vi "HideUnusedControls.vi"(11 "AllControlsRefs":T22) -> ()   [LabVIEW 2013]
uses:
  <instrlib>/DG535/Command/DG535_TriggerMode.ctl
  <instrlib>/DG535/SRS_DG535_Lib.lvlib
  <instrlib>/DG535/Command/DG535_Output.ctl
  <instrlib>/DG535/Command/DG535_Channel.ctl
  <instrlib>/DG535/Command/Set Output.ctl
  <instrlib>/DG535/Command/Set Delay.ctl
  <instrlib>/DG535/Command/Set Trigger.ctl
  ControlDef/AllControlsRefs.ctl
  ControlDef/ProcessingMode.ctl
  <instrlib>/AnalogDiscSDKLv/VIs/DWF_TrigSrc.ctl
  <instrlib>/AnalogDiscSDKLv/AnalogDiscSDKLv.lvlib
  <instrlib>/AnalogDiscSDKLv/VIs/DWF_Filter.ctl
  <instrlib>/AnalogDiscSDKLv/VIs/DWF_AcqMode.ctl
  <instrlib>/AnalogDiscSDKLv/VIs/DWF_TrigCond.ctl
  <instrlib>/AnalogDiscSDKLv/VIs/DWF_TrigType.ctl
  <instrlib>/AnalogDiscSDKLv/VIs/DWF_AnalogIn_Configurations.ctl
  <instrlib>/GageLv_uic/VI/Gage_Configs.ctl
  <instrlib>/GageLv_uic/Gage.lvlib
  ControlDef/InstruMode_Typedef.ctl
  ControlDef/LaserCtrl_Method.ctl
  ControlDef/MainDAQ_Selector.ctl
panel:
  in  "InstruConfig":T18 {"DG535"."Trigger"."External  Level" min=-2.56 max=2.56 format="%.2f"; "DG535"."Trigger"."Internal/Burst Rate" min=0.001 max=1000000.0 format="%.3f"; "DG535"."Delays"."Delay" format="%#_6p"; "DG535"."Output"."Offset" min=-3.0 max=4.0 format="%.2f"; "DG535"."Output"."Amplitude" min=-3.0 max=4.0 format="%.2f"; "Gage_Config"."Trigger"."External Impedance" items=["50 Ohm", "HiZ"]; "Gage_Config"."Trigger"."External Coupling" items=["DC", "AC"]; "Gage_Config"."Trigger"."External Range" min=2000 max=10000 step=8000; "Gage_Config"."Trigger"."Slope" items=["Rising", "Falling"]; "Gage_Config"."Trigger"."Level" min=-100 max=100; "Gage_Config"."Trigger"."Source" min=0 max=64 step=1; "Gage_Config"."Channels"."Impedance" min=50 max=1000000 step=999950; "Gage_Config"."Channels"."Coupling" items=["DC", "AC"]; "Gage_Config"."Acquisition"."Segment Size" min=256.0 step=128.0; "Gage_Config"."Acquisition"."Trigger Delay" min=0.0 step=128.0; "Gage_Config"."Acquisition"."Trigger Timeout" format="%.0p"; "Gage_Config"."Acquisition"."Trigger Holdoff" min=0.0 step=128.0; "Gage_Config"."Acquisition"."Depth" min=256.0 step=128.0; "Gage_Config"."Acquisition"."Mode" items=["Single", "Dual", "Quad", "Octal"]; "Gage_Config"."Acquisition"."Sample Rate" format="%.0p"; "AnalogDisc_Config"."AnalogTrigger"."Level(V)" format="%#_6p"; "AnalogDisc_Config"."AnalogTrigger"."Hysterisis(V)" format="%#_6p"; "AnalogDisc_Config"."Acqusition"."RecordLength(s)" format="%#_6p"; "AnalogDisc_Config"."Acqusition"."Freq(Hz,SampleRate)" format="%#_6p"; "AnalogDisc_Config"."Trigger"."Position/Delay(s)" format="%#_6p"; "AnalogDisc_Config"."Trigger"."Holdoff(s)" format="%#_6p"; "AnalogDisc_Config"."Trigger"."Timeout(s)" format="%#_6p"}
  in  "DG535_Configs":T19={"Trigger"={"Trigger Mode"=enum."External", "Internal/Burst Rate"=10.0, "External  Level"=1.5, "Impedance"=TRUE, "Slope"=FALSE}, "Delays"=[{"Channel"=enum."A Output", "Sync To"=enum."T0 Output", "Delay"=0.099807701}, {"Channel"=enum."B Output", "Sync To"=enum."A Output", "Delay"=1.2e-05}, {"Channel"=enum."C Output", "Sync To"=enum."T0 Output", "Delay"=0.0}, {"Channel"=enum."D Output", "Sync To"=enum."T0 Output", "Delay"=1e-05}, {"Channel"=enum."Trigger Input", "Sync To"=enum."T0 Output", "Delay"=0.0}], "Output"=[{"Channel"=enum."A Output", "Level"=enum."TTL", "Load"=TRUE, "Polarity"=FALSE, "Amplitude"=1.0, "Offset"=0.0}, {"Channel"=enum."B Output", "Level"=enum."TTL", "Load"=FALSE, "Polarity"=TRUE, "Amplitude"=1.0, "Offset"=0.0}, {"Channel"=enum."C Output", "Level"=enum."TTL", "Load"=TRUE, "Polarity"=FALSE, "Amplitude"=1.0, "Offset"=0.0}, {"Channel"=enum."D Output", "Level"=enum."TTL", "Load"=TRUE, "Polarity"=FALSE, "Amplitude"=1.0, "Offset"=0.0}, {"Channel"=enum."T0 Output", "Level"=enum."TTL", "Load"=FALSE, "Polarity"=FALSE, "Amplitude"=1.0, "Offset"=0.0}, {"Channel"=enum."AB Output", "Level"=enum."TTL", "Load"=TRUE, "Polarity"=FALSE, "Amplitude"=1.0, "Offset"=0.0}, {"Channel"=enum."CD Output", "Level"=enum."TTL", "Load"=TRUE, "Polarity"=FALSE, "Amplitude"=1.0, "Offset"=0.0}]} caption="DG535 Settings (Restart Needed)" {"Trigger"."External  Level" min=-2.56 max=2.56 format="%.2f"; "Trigger"."Internal/Burst Rate" min=0.001 max=1000000.0 format="%.3f"; "Delays"."Delay" format="%#_6p"; "Output"."Offset" min=-3.0 max=4.0 format="%.2f"; "Output"."Amplitude" min=-3.0 max=4.0 format="%.2f"}
  in  "SRS On/Off":bool caption="Dont Rely On\nShowing\nCheck BNC"
  in  "Internal/Burst Rate":dbl=10.0 caption="Internal/Burst Rate (Hz)" min=0.001 max=1000000.0 format="%.3f"
  in  "Trigger Mode (SRS)":T5=enum."External" caption="Trigger Mode"
  in  "Ch_D":dbl=2.8e-05 format="%_3ps"
  in  "Ch_C":dbl format="%_3ps"
  in  "Ch_B":dbl=3e-05 format="%_3ps"
  in  "Ch_A":dbl=0.099807701 format="%_3ps"
  in  "Delay A":dbl format="%_3ps"
  in  "Width B":dbl=1e-06 min=0.0 max=9.9e-05 step=1e-09 format="%_3ps"
  in  "Width A":dbl=1e-06 min=0.0 max=9.9e-05 step=1e-09 format="%_3ps"
  in  "Delay B":dbl min=0.0 max=9.9e-05 step=1e-09 format="%_3ps"
  in  "Rep.Rate (BNC)":dbl=10.0 caption="Repetive Rate" min=0.0 max=1000.0 format="%#_6f Hz"
  in  "Mode (BNC)":T20(ring)=enum."Single Shot" caption="Mode"
  in  "Channels Enable Status":bool[](array[boolean])=[TRUE, TRUE]
  in  "Trigger Mode (BNC)":T21(ring)=enum."Triggered" caption="Trigger Mode"
  in  "BNC On/Off":bool caption="Dont Rely On\nShowing\nCheck BNC"
  in  "ManlTrig(SDG)":bool caption="Manual Trigger"
  in  "Mode(SDG_II)":bool caption="Mode"
  in  "Switch(SDG_II)":bool caption="Status"
  out "Nd:YAG Energy":dbl(slide) caption="Nd:YAG Energy (J)" scale=0.0..0.03 scale format="%#_2p"
  out "High Voltages":T23 {"Einzel (Source)" format="%#.0f"; "Einzel (TOF)" format="%#.0f"; "Cone" format="%#.0f"}
  out "LaserEnergy":dbl(slide) caption="Spitfire Energy (J)" scale=0.0..2e-06 scale format="%#_2p"
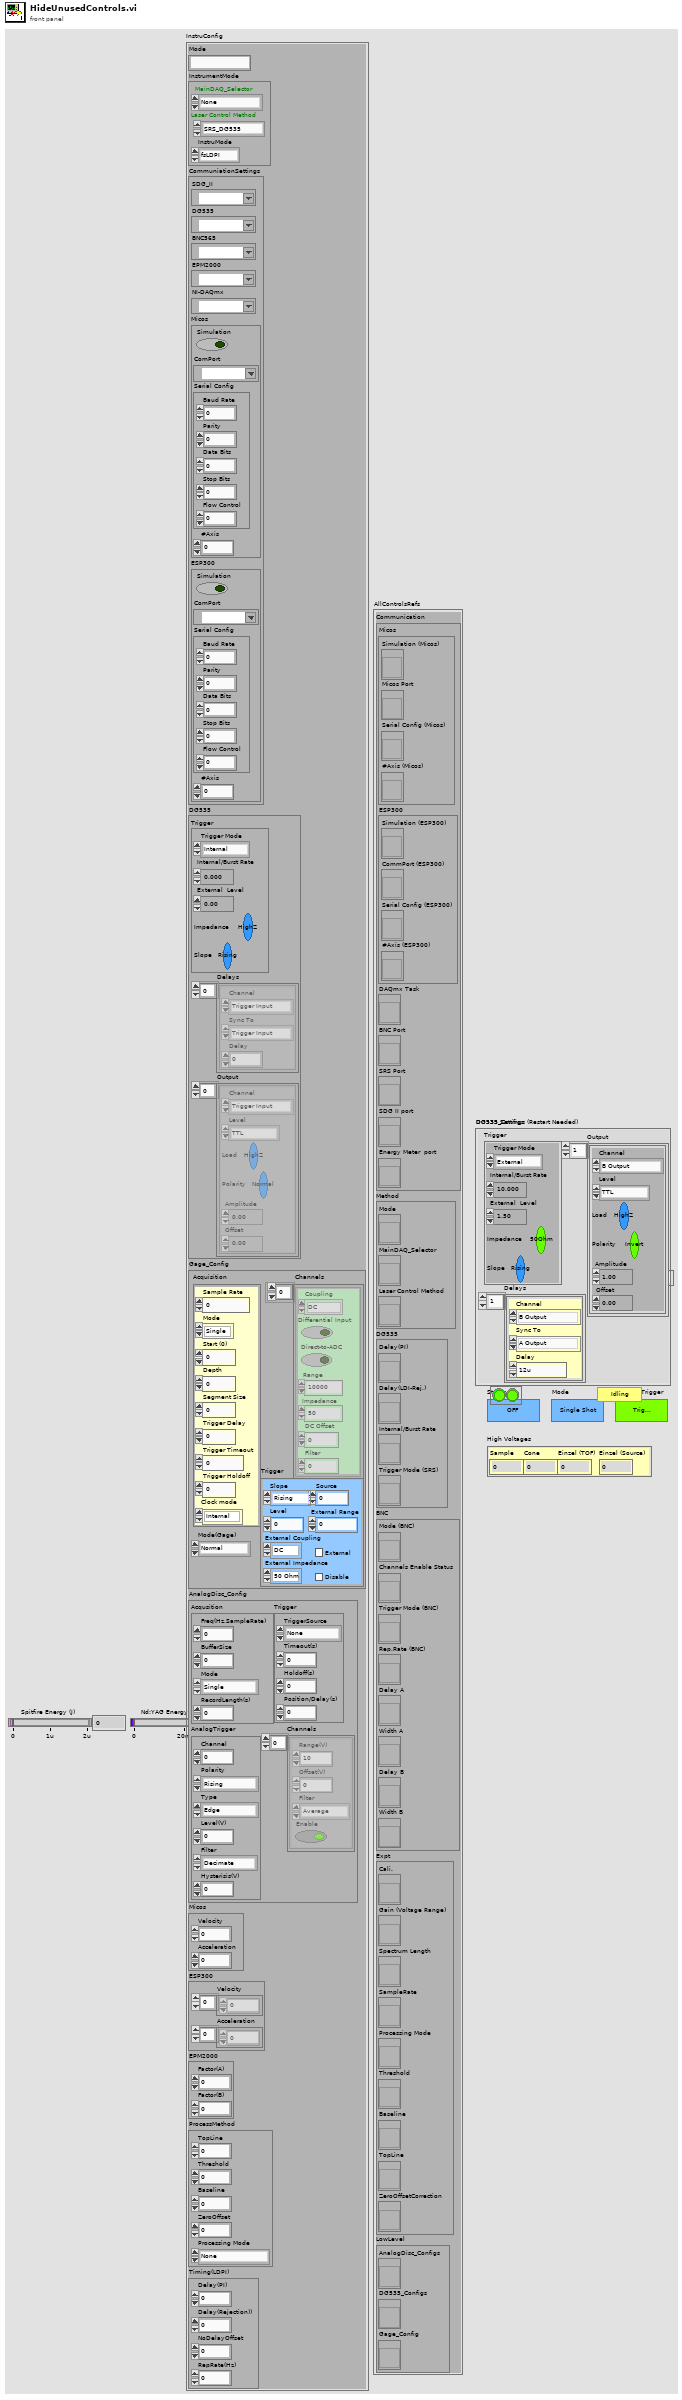
[diagram p1: front panel]
types:
  T1 = typedef "MainDAQ_Selector.ctl" = enum16{"None", "Gage", "Gage_Double", "IonWerks_TDCx4", "Tektronics", "KnifeEdge_Emu", "AnalogDisc"}
  T2 = typedef "LaserCtrl_Method.ctl" = enum16{"SRS_DG535", "BNC", "SDG_II"}
  T3 = typedef "InstruMode_Typedef.ctl" = enum16{"fsLDPI", "nsLDPI", "nsLD-fsPI", "GenericTOF", "BeamProfiling"}
  T4 = typedef "SRS_DG535_Lib.lvlib/Set Trigger.ctl" = cluster{"Trigger Mode":T5, "Internal/Burst Rate":dbl, "External  Level":sgl, "Impedance":bool, "Slope":bool}
  T5 = typedef "SRS_DG535_Lib.lvlib/DG535_TriggerMode.ctl" = enum16{"Internal", "External", "SingleShot", "Burst", "Line"}
  T6 = typedef "SRS_DG535_Lib.lvlib/Set Delay.ctl" = cluster{"Channel":T7, "Sync To":T7, "Delay":dbl}
  T7 = typedef "SRS_DG535_Lib.lvlib/DG535_Channel.ctl" = enum16{"Trigger Input", "T0 Output", "A Output", "B Output", "AB Output", "C Output", "D Output", "CD Output", "NULL"}
  T8 = typedef "SRS_DG535_Lib.lvlib/Set Output.ctl" = cluster{"Channel":T7, "Level":T9, "Load":bool, "Polarity":bool, "Amplitude":dbl, "Offset":dbl}
  T9 = typedef "SRS_DG535_Lib.lvlib/DG535_Output.ctl" = enum16{"TTL", "NIM", "ECL", "Variable"}
  T10 = typedef "Gage.lvlib/Gage_Configs.ctl" = cluster{"Acquisition":cluster{"Sample Rate":dbl, "Mode":u16, "Start (0)":dbl, "Depth":dbl, "Segment Size":dbl, "Trigger Delay":dbl, "Trigger Timeout":dbl, "Trigger Holdoff":dbl, "Clock mode":enum16{"Internal", "External", "Reference"}}, "Channels":cluster{"Coupling":u16, "Differential Input":bool, "Direct-to-ADC":bool, "Range":u32, "Impedance":u32, "DC Offset":i32, "Filter":i32}[], "Trigger":cluster{"Slope":u16, "Level":i32, "Source":i32, "External Range":u32, "External Coupling":u16, "External":bool, "Disable":bool, "External Impedance":u16}, "Mode(Gage)":enum16{"Normal", "Continuous", "MultiRecord", "HwAverage"}}
  T11 = typedef "AnalogDiscSDKLv.lvlib/DWF_AnalogIn_Configurations.ctl" = cluster{"Acqusition":cluster{"Freq(Hz,SampleRate)":dbl, "BufferSize":i32, "Mode":T12, "RecordLength(s)":dbl}, "Channels":cluster{"Range(V)":dbl, "Offset(V)":dbl, "Filter":T13, "Enable":bool}[], "Trigger":cluster{"TriggerSource":T14, "Timeout(s)":dbl, "Holdoff(s)":dbl, "Position/Delay(s)":dbl}, "AnalogTrigger":cluster{"Channel":i32, "Polarity":T15, "Type":T16, "Level(V)":dbl, "Filter":T13, "Hysterisis(V)":dbl}}
  T12 = typedef "AnalogDiscSDKLv.lvlib/DWF_AcqMode.ctl" = enum16{"Single", "ScanShift", "ScanScreen", "Record"}
  T13 = typedef "AnalogDiscSDKLv.lvlib/DWF_Filter.ctl" = enum16{"Decimate", "Average", "MinMax"}
  T14 = typedef "AnalogDiscSDKLv.lvlib/DWF_TrigSrc.ctl" = enum16{"None", "PC", "DetectorAnalogIn", "DetectorDigitalIn", "AnalogIn", "DigitalIn", "DigitalOut", "AnalogOut1", "AnalogOut2", "AnalogOut3", "AnalogOut4", "External1", "External2", "External3", "External4"}
  T15 = typedef "AnalogDiscSDKLv.lvlib/DWF_TrigCond.ctl" = enum16{"Rising", "Falling"}
  T16 = typedef "AnalogDiscSDKLv.lvlib/DWF_TrigType.ctl" = enum16{"Edge", "Pulse", "Transition"}
  T17 = typedef "ProcessingMode.ctl" = enum16{"None", "Drop by Threshold", "TDC Simulate", "SetFilter"}
  T18 = cluster{"Mode":string, "InstrumentMode":cluster{"MainDAQ_Selector":T1, "Laser Control Method":T2, "InstruMode":T3}, "CommuniationSettings":cluster{"SDG_II":refnum<visa-resource-name>, "DG535":refnum<visa-resource-name>, "BNC565":refnum<visa-resource-name>, "EPM2000":refnum<visa-resource-name>, "NI-DAQmx":refnum<visa-resource-name>, "Micos":cluster{"Simulation":bool, "ComPort":refnum<visa-resource-name>, "Serial Config":cluster{"Baud Rate":u32, "Parity":u16, "Data Bits":u16, "Stop Bits":u16, "Flow Control":u16}, "#Axis":i32}, "ESP300":cluster{"Simulation":bool, "ComPort":refnum<visa-resource-name>, "Serial Config":cluster{"Baud Rate":u32, "Parity":u16, "Data Bits":u16, "Stop Bits":u16, "Flow Control":u16}, "#Axis":i32}}, "DG535":cluster{"Trigger":T4, "Delays":T6[], "Output":T8[]}, "Gage_Config":T10, "AnalogDisc_Config":T11, "Micos":cluster{"Velocity":dbl, "Acceleration":dbl}, "ESP300":cluster{"Velocity":dbl[], "Acceleration":dbl[]}, "EPM2000":cluster{"Factor(A)":dbl, "Factor(B)":dbl}, "ProcessMethod":cluster{"TopLine":dbl, "Threshold":dbl, "Baseline":dbl, "ZeroOffset":dbl, "Processing Mode":T17}, "Timing(LDPI)":cluster{"Delay(PI)":dbl, "Delay(Rejection))":dbl, "NoDelayOffset":dbl, "RepRate(Hz)":dbl}}
  T19 = cluster{"Trigger":T4, "Delays":T6[], "Output":T8[]}
  T20 = enum16{"Normal", "Single Shot", "Duty Cycle", "Burst"}
  T21 = enum16{"Disabled", "Triggered", "Gated", "Triggered & Gated"}
  T22 = typedef "AllControlsRefs.ctl" = cluster{"Communication":cluster{"Micos":cluster{"Simulation (Micos)":refnum<vi>, "Micos Port":refnum<vi>, "Serial Config (Micos)":refnum<vi>, "#Axis (Micos)":refnum<vi>}, "ESP300":cluster{"Simulation (ESP300)":refnum<vi>, "CommPort (ESP300)":refnum<vi>, "Serial Config (ESP300)":refnum<vi>, "#Axis (ESP300)":refnum<vi>}, "DAQmx Task":refnum<vi>, "BNC Port":refnum<vi>, "SRS Port":refnum<vi>, "SDG II port":refnum<vi>, "Energy Meter  port":refnum<vi>}, "Method":cluster{"Mode":refnum<vi>, "MainDAQ_Selector":refnum<vi>, "Laser Control Method":refnum<vi>}, "DG535":cluster{"Delay(PI)":refnum<vi>, "Delay(LDI-Rej.)":refnum<vi>, "Internal/Burst Rate":refnum<vi>, "Trigger Mode (SRS)":refnum<vi>}, "BNC":cluster{"Mode (BNC)":refnum<vi>, "Channels Enable Status":refnum<vi>, "Trigger Mode (BNC)":refnum<vi>, "Rep.Rate (BNC)":refnum<vi>, "Delay A":refnum<vi>, "Width A":refnum<vi>, "Delay B":refnum<vi>, "Width B":refnum<vi>}, "Expt":cluster{"Cali.":refnum<vi>, "Gain (Voltage Range)":refnum<vi>, "Spectrum Length":refnum<vi>, "SampleRate":refnum<vi>, "Processing Mode":refnum<vi>, "Threshold":refnum<vi>, "Baseline":refnum<vi>, "TopLine":refnum<vi>, "ZeroOffsetCorrection":refnum<vi>}, "LowLevel":cluster{"AnalogDisc_Configs":refnum<vi>, "DG535_Configs":refnum<vi>, "Gage_Config":refnum<vi>}}
  T23 = cluster{"Sample":dbl, "Cone":dbl, "Einzel (TOF)":dbl, "Einzel (Source)":dbl}
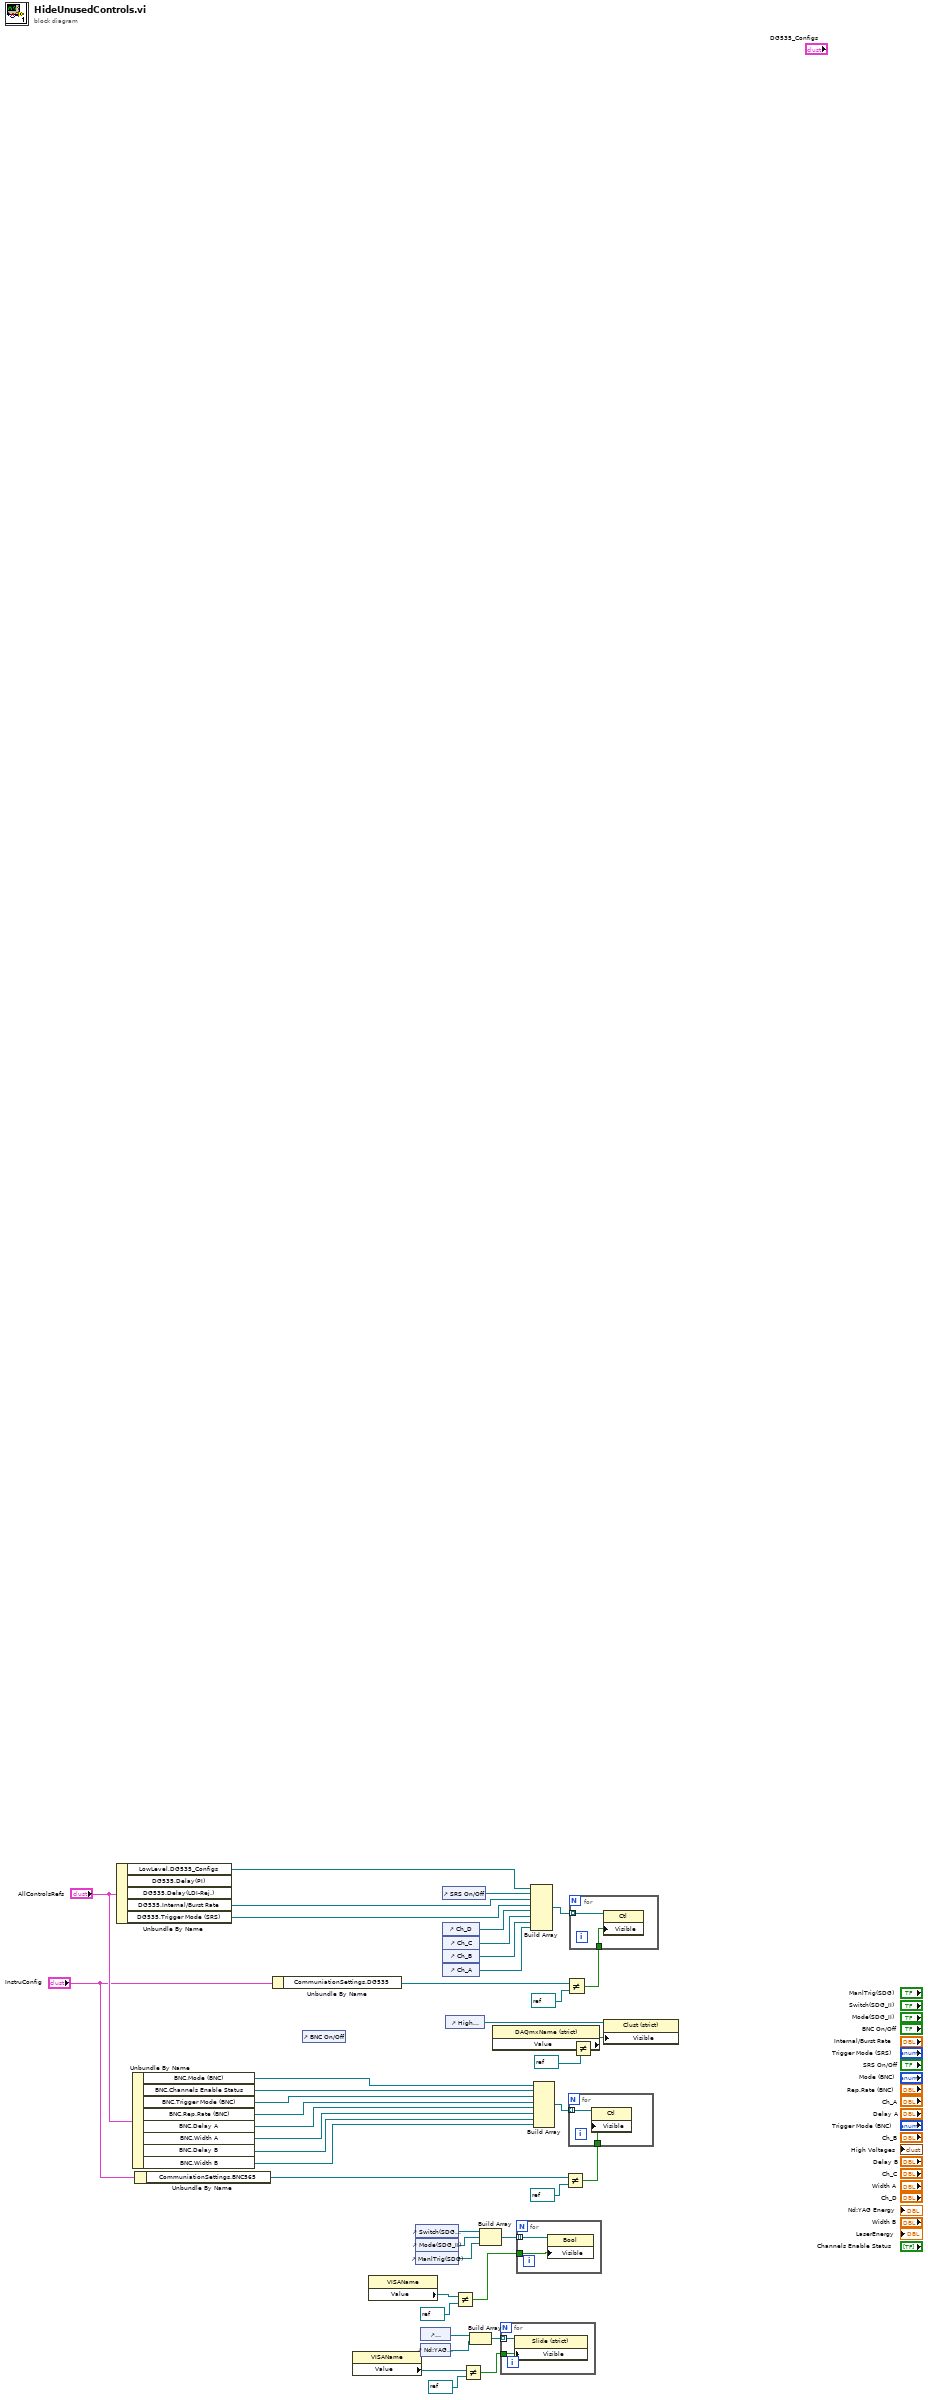
[diagram p0: block diagram]
diagram:
  n1 = Unbundle By Name("AllControlsRefs") -> ("LowLevel.DG535_Configs"=w13:refnum<vi>, "DG535.Internal/Burst Rate"=w15:refnum<vi>, "DG535.Trigger Mode (SRS)"=w14:refnum<vi>)  [unwired: 2 out]
  n2 = Unbundle By Name("AllControlsRefs") -> ("BNC.Mode (BNC)"=w10:refnum<vi>, "BNC.Channels Enable Status"=w9:refnum<vi>, "BNC.Trigger Mode (BNC)"=w8:refnum<vi>, "BNC.Rep.Rate (BNC)"=w7:refnum<vi>, "BNC.Delay A"=w6:refnum<vi>, "BNC.Width A"=w5:refnum<vi>, "BNC.Delay B"=w4:refnum<vi>, "BNC.Width B"=w3:refnum<vi>)
  n3 = Unbundle By Name("InstruConfig") -> ("CommuniationSettings.BNC565"=w1:refnum<visa-resource-name>)
  n4 = Unbundle By Name("InstruConfig") -> ("CommuniationSettings.DG535"=w12:refnum<visa-resource-name>)
  n5 = control-ref of="BNC On/Off"() -> ()  [unwired: 1 out]
  n6 = property on="Property Node" class="VISAName"() -> ("Value"=w28:refnum<visa-resource-name>)  [unwired: 2 in, 2 out]
  n7 = property on="Property Node" class="VISAName"() -> ("Value"=w25:refnum<visa-resource-name>)  [unwired: 2 in, 2 out]
  n8 = control-ref of="Switch(SDG_II)"() -> (w19:refnum<vi>)
  n9 = control-ref of="Mode(SDG_II)"() -> (w20:refnum<vi>)
  n10 = control-ref of="ManlTrig(SDG)"() -> (w21:refnum<vi>)
  n11 = control-ref of="LaserEnergy"() -> (w29:refnum<vi>)
  n12 = control-ref of="Nd:YAG Energy"() -> (w30:refnum<vi>)
  n13 = control-ref of="SRS On/Off"() -> (w43:refnum<vi>)
  n14 = control-ref of="Ch_D"() -> (w42:refnum<vi>)
  n15 = control-ref of="Ch_C"() -> (w41:refnum<vi>)
  n16 = control-ref of="Ch_B"() -> (w40:refnum<vi>)
  n17 = control-ref of="Ch_A"() -> (w39:refnum<vi>)
  n18 = control-ref of="High Voltages"() -> (w35:refnum<vi>)
  n19 = Not Equal?(x=w25, y=refnum<visa-resource-name> refnum ("BNC Port")) -> (x != y?=w22:bool)
  n20 = Not Equal?(x=w28, y=refnum<visa-resource-name> refnum ("BNC Port")) -> (x != y?=w26:bool)
  n21 = Build Array(w29, w30) -> (w31:refnum<vi>[])
  n22 = Build Array(w19, w20, w21) -> (w24:refnum<vi>[])
  n23 = property on="Property Node" class="DAQmxName (strict)"() -> ("Value"=w34:refnum<k21>)  [unwired: 2 in, 2 out]
  n24 = for {
    tunnel: w31 -> [w45] mode=indexing
    tunnel: w26 -> [w44]
    n25 = property class="Slide (strict)"(reference=w45, "Visible"=w44) -> ()  [unwired: 1 in, 2 out]
  }
  n26 = for {
    tunnel: w24 -> [w47] mode=indexing
    tunnel: w22 -> [w46]
    n27 = property class="Bool"(reference=w47, "Visible"=w46) -> ()  [unwired: 1 in, 2 out]
  }
  n28 = Build Array(w13, w43, w15, w14, w42, w41, w40, w39) -> (w36:refnum<vi>[])
  n29 = Build Array(w10, w9, w8, w7, w6, w5, w4, w3) -> (w16:refnum<vi>[])
  n30 = Not Equal?(x=w1, y=refnum<visa-resource-name> refnum ("BNC Port")) -> (x != y?=w18:bool)
  n31 = Not Equal?(x=w12, y=refnum<visa-resource-name> refnum ("BNC Port")) -> (x != y?=w38:bool)
  n32 = for {
    tunnel: w16 -> [w49] mode=indexing
    tunnel: w18 -> [w48]
    n33 = property class="Ctl"(reference=w49, "Visible"=w48) -> ()  [unwired: 1 in, 2 out]
  }
  n34 = for {
    tunnel: w36 -> [w51] mode=indexing
    tunnel: w38 -> [w50]
    n35 = property class="Ctl"(reference=w51, "Visible"=w50) -> ()  [unwired: 1 in, 2 out]
  }
  n36 = Not Equal?(x=w34, y=refnum<k21> refnum) -> (x != y?=w33:bool)
  n37 = property class="Clust (strict)"(reference=w35, "Visible"=w33) -> ()  [unwired: 1 in, 2 out]
